vi "Move Home Impl.vi"(8 "error in (no error)":errorcluster, 11 "ASI Stage in":refnum<class "ASI Stage.lvclass">) -> (0 "error out":errorcluster, 3 "ASI Stage out":refnum<class "ASI Stage.lvclass">)   [LabVIEW 2023, in "ASI Stage.lvlib" / "ASI Stage.lvclass"]
uses:
  ASI Stage.lvclass
  ASI Stage.lvclass/ASI Stage.ctl
  <instrlib>/ASI TG-1000/ASI TG-1000.lvlib
  <instrlib>/ASI TG-1000/Public/Utility/Axis Name.ctl
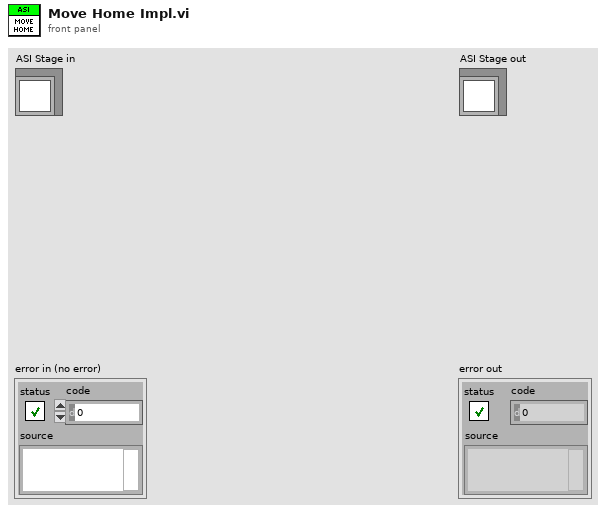
[diagram p1: front panel]
types:
  T1 = typedef "ASI TG-1000.lvlib/Axis Name.ctl" = enum8{"undefined", "A", "B", "C", "D", "E", "F", "G", "H", "I", "J", "K", "L", "M", "N", "O", "P", "Q", "R", "S", "T", "U", "V", "W", "X", "Y", "Z"}
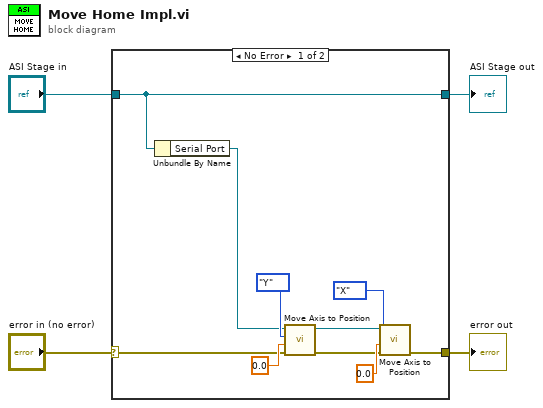
[diagram p0: block diagram]
diagram:
  n1 = case shown="No Error" "error in (no error)" {
    selector: "error in (no error)" -> [w9 w15]
    tunnel: [w7 w15] -> w3
    tunnel: "ASI Stage in" -> [w6 w16]
    tunnel: [w6 w16] -> w1
    frame No Error {
      n2 = Unbundle By Name(w6) -> ("Serial Port"=w5:refnum<visa-resource-name>)
      n3 = call <instrlib>:"Move Axis to Position.vi"("error in (no error)"=w9, "Position [internal units]"=0.0, "Axis"=Axis_Name."Y", "VISA in"=w5) -> ("error out"=w8:errorcluster, "VISA out"=w12:refnum<visa-resource-name>)  [unwired: 5 in]
      n4 = call <instrlib>:"Move Axis to Position.vi"("error in (no error)"=w8, "Position [internal units]"=0.0, "Axis"=Axis_Name."X", "VISA in"=w12) -> ("error out"=w7:errorcluster)  [unwired: 5 in, 1 out]
    }
    frame Error {
    }
  }
  "error out" <- w3
  "ASI Stage out" <- w1
